vi "WRP Get Kinetic Energy.vi"(8 "error in (no error)":errorcluster) -> (0 "error out":errorcluster, 2 "function return":i32, 3 "kinetic_energy":dbl)   [LabVIEW 2018, in "SesWrapper.lvlib"]
doc: "int STDCALL WRP_GetKineticEnergy(double *kinetic_energy);"
uses:
  SesWrapper.lvlib
  build/Debug/SESWrapper.dll
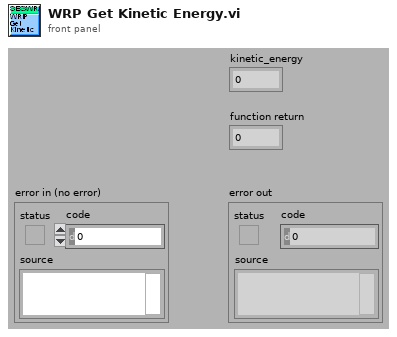
[diagram p1: front panel]
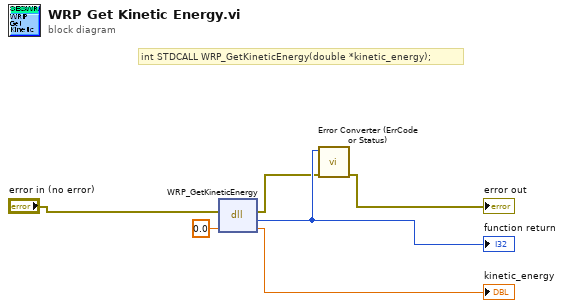
[diagram p0: block diagram]
diagram:
  # "int STDCALL WRP_GetKineticEnergy(double *kinetic_energy);"
  n1 = dll-call lib="C:/Development/svn/seswrapper-lib/build/Debug/SESWrapper.*" fn="WRP_GetKineticEnergy"(error in="error in (no error)", "kinetic_energy"=0.0) -> (error out=w2:errorcluster, w6:i32, "kinetic_energy"=→"kinetic_energy":dbl)  [unwired: 2 in, 1 out]
  "function return" <- w6
  n2 = call "Error Converter (ErrCode or Status).vi"("error in (no error)"=w2, "error code"=w6) -> ("error out"=→"error out":errorcluster)  [unwired: 9 in]
